vi "실습 5-5.vi"() -> ()   [LabVIEW 2014]
panel:
  out "에러 출력":errorcluster
  out "웨이브폼 그래프":waveform(dbl)(graph)
  in  "amplitude":dbl
  in  "signal type":T1(ring)
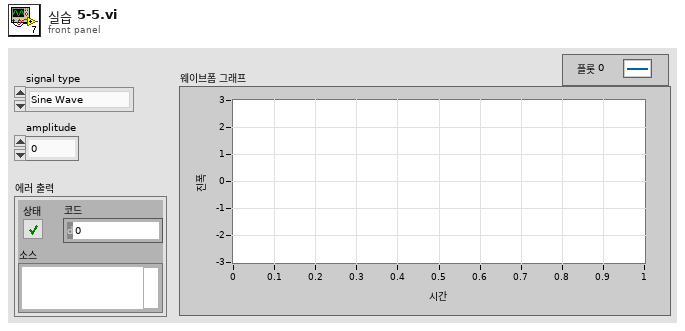
[diagram p1: front panel]
types:
  T1 = enum16{"Sine Wave", "Triangle Wave", "Square Wave", "Sawtooth Wave"}
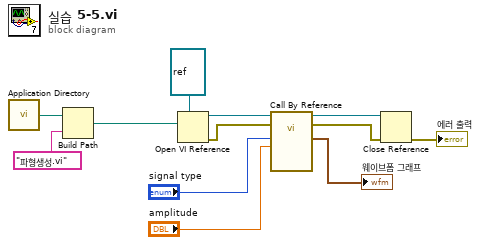
[diagram p0: block diagram]
diagram:
  n1 = call <vilib>:"Application Directory.vi"() -> ("Application Directory"=w4:path)
  n2 = Build Path(base path=w4, name or relative path="파형생성.vi" ("이름 또는 상대 경로")) -> (appended path=w2:path)
  n3 = Open VI Reference(type specifier VI Refnum (for type only)=refnum<vi> refnum ("타입 지정자 VI 참조 번호(타입만)"), vi path=w2) -> (vi reference=w11:refnum<vi>, error out=w10:errorcluster)  [unwired: 4 in]
  n4 = call-by-ref "?"(reference=w11, error in=w10, "amplitude"="amplitude", "signal type"="signal type") -> (reference out=w9:refnum<vi>, error out=w8:errorcluster, "웨이브폼 그래프"=→"웨이브폼 그래프":waveform(dbl))  [unwired: 9 in]
  n5 = Close Reference(reference=w9, error in (no error)=w8) -> (error out=→"에러 출력":errorcluster)
